vi "Periodic Message Filter.vi"(5 "Remove Immediately?(F)":bool, 7 "reset?":bool, 8 "Settings":T1={"threashold(#/s)"=1.0, "Check Peroid(s)"=1.0}, 11 "Cross CSM Data":T2={"Name(\"\" to use uuid)"="CSM Tiny", "Current State"="UI: Refresh Buttons", "Arguments"="", "Source Message"={"‘State"="", "’Arguments"="", "’Error"={"status"=FALSE, "code"=0, "source"=""}}, "Source Module"="<end>", "Complete(T)/Start(F)"=TRUE, "LogType"=enum."State Change"}) -> (0 "Boolean":bool, 1 "filter Strings Count":string[](array[string]), 3 "Log String":string)   [LabVIEW 2017, in "csm-tool-support.lvlib"]
uses:
  csm-tool-support.lvlib
  _Support/Typedef/_CSM_GlobalLog_MSG.ctl
  _Support/Typedef/_CSM_Response Source Message.ctl
  _Support/Typedef/_CSM_GlobalLog_MSG_TYPE.ctl
  Communicable State Machine.lvlib
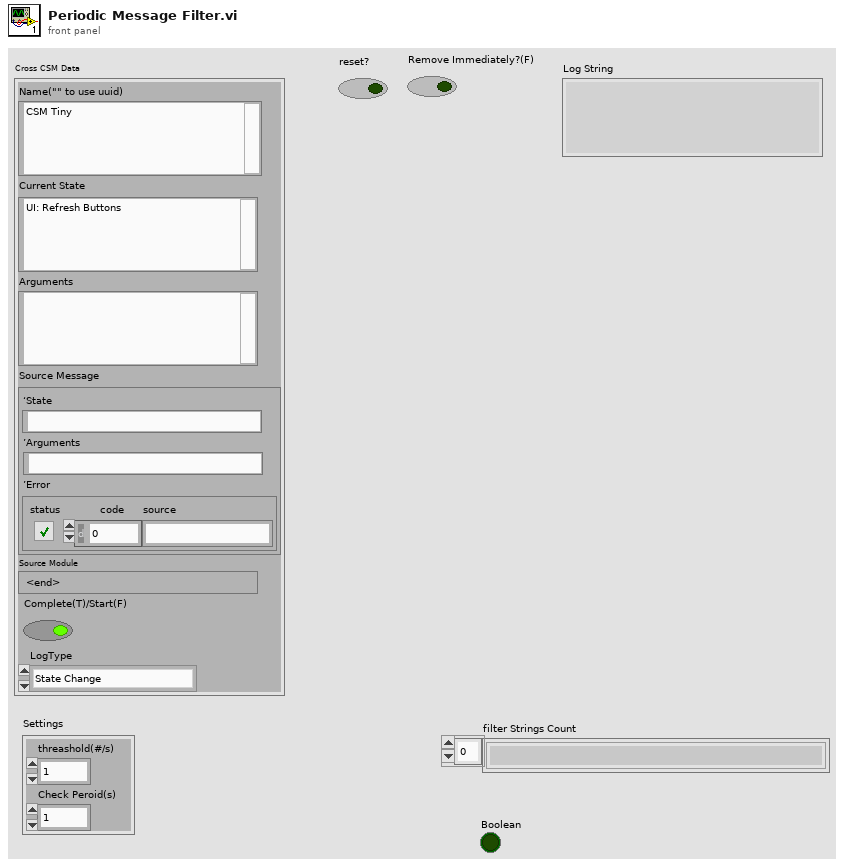
[diagram p1: front panel]
types:
  T1 = cluster{"threashold(#/s)":dbl, "Check Peroid(s)":dbl}
  T2 = typedef "Communicable State Machine.lvlib/_CSM_GlobalLog_MSG.ctl" = cluster{"Name(\"\" to use uuid)":string, "Current State":string, "Arguments":string, "Source Message":T3, "Source Module":string, "Complete(T)/Start(F)":bool, "LogType":T4}
  T3 = typedef "Communicable State Machine.lvlib/_CSM_Response Source Message.ctl" = cluster{"‘State":string, "’Arguments":string, "’Error":errorcluster}
  T4 = typedef "Communicable State Machine.lvlib/_CSM_GlobalLog_MSG_TYPE.ctl" = enum16{"User Log", "State Change", "Status", "Interrupt", "Register", "Unregister", "Error Log", "Module Created", "Module Destroyed"}
  T5 = cluster{"String":string, "Count":i64, "since":timestamp}[]
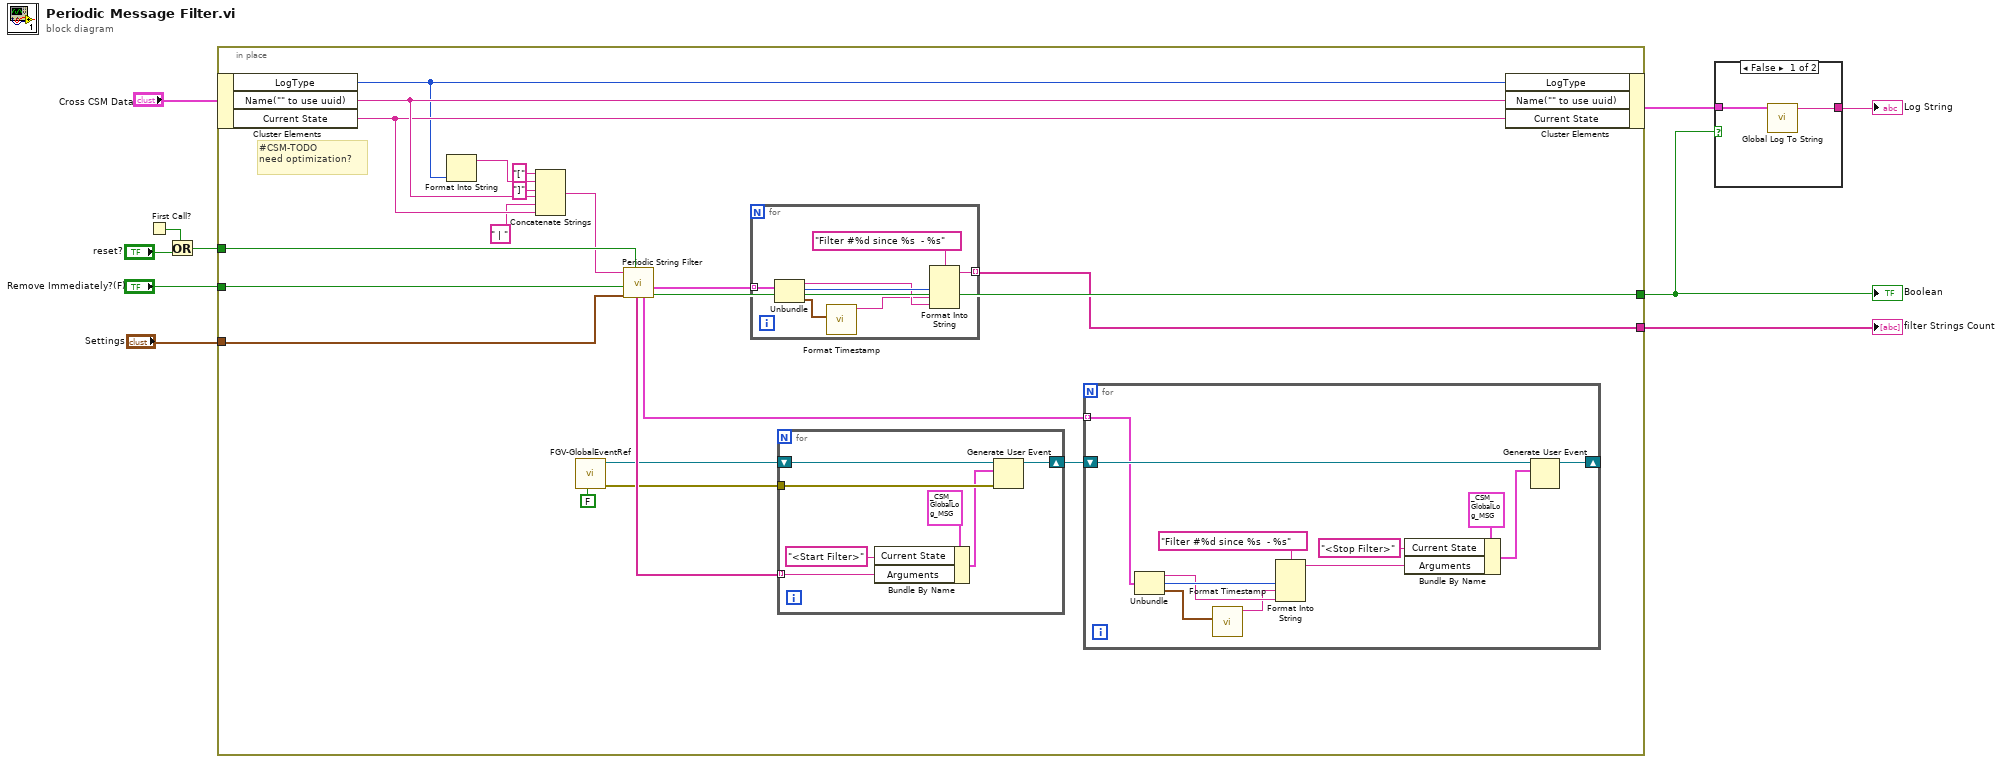
[diagram p0: block diagram]
diagram:
  n1 = First Call?() -> (First Call?: T/F=w7:bool)
  n2 = Or(x=w7, y="reset?") -> (x .or. y?=w5:bool)
  n3 = in-place {
    in-place-border: w5 -> [w25]
    in-place-border: [w23] -> w4
    in-place-border: [w19] -> w3
    in-place-border: "Remove Immediately?(F)" -> [w12]
    in-place-border: "Settings" -> [w11]
    # "#CSM-TODO\nneed optimization?"
    n4 = in-place-cluster #1("Cross CSM Data") -> ("LogType"=w28:T4, "Name(\"\" to use uuid)"=w30:string, "Current State"=w29:string)
    n5 = Format Into String(w28) -> (resulting string=w27:string)  [unwired: 3 in, 1 out]
    n6 = Concatenate Strings("[" ("string"), w27, "]" ("string"), w30, " | " ("string"), w29) -> (w24:string)
    n7 = call "FGV-GlobalEventRef.vi"("Create(F)"=FALSE) -> ("error out"=w15:errorcluster, "CSM Global Log Event"=w16:refnum<user-event>)  [unwired: 9 in]
    n8 = call "Periodic String Filter.vi"("reset?"=w25, "Settings"=w11, "Remove Immediately?(F)"=w12, "Input String"=w24) -> ("filtered?"=w23:bool, "Filtered Status"=w20:T5, "removed info"=w13:T5, "added Info"=w18:string[])  [unwired: 3 in, 1 out]
    n9 = for {
      tunnel: w20 -> [w55] mode=indexing
      tunnel: [w56] -> w19 mode=indexing
      n10 = Unbundle(w55) -> ("String"=w53:string, "Count"=w54:i64, "since"=w51:timestamp)
      n11 = call "Format Timestamp.vi"("timestamp"=w51) -> ("String"=w50:string)  [unwired: 10 in]
      n12 = Format Into String(format string="Filter #%d since %s  - %s", w54, w50, w53) -> (resulting string=w56:string)  [unwired: 2 in, 1 out]
    }
    n13 = for {
      tunnel: w18 -> [w44] mode=indexing
      tunnel: w15 -> [w48]
      shift-right: [w47] -> w14
      shift-left: w16 -> [w49]
      n14 = Bundle By Name(cluster=T2 {"Name(\"\" to use uuid)"="", "Current State"="", "Arguments"="", "Source Message"={"‘State"="", "’Arguments"="", "’Error"={"status"=FALSE, "code"=0, "source"=""}}, "Source Module"="", "Complete(T)/Start(F)"=FALSE, "LogType"=enum."User Log"} ("event data"), "Current State"="<Start Filter>", "Arguments"=w44) -> (w45:T2)
      n15 = Generate User Event(user event=w49, event data cluster=w45, error in=w48) -> (user event out=w47:refnum<user-event>)  [unwired: 1 in, 1 out]
    }
    n16 = for {
      shift-right: [w41] -> _
      shift-left: w14 -> [w42]
      tunnel: w13 -> [w37] mode=indexing
      n17 = Unbundle(w37) -> ("String"=w33:string, "Count"=w34:i64, "since"=w32:timestamp)
      n18 = call "Format Timestamp.vi"("timestamp"=w32) -> ("String"=w31:string)  [unwired: 10 in]
      n19 = Format Into String(format string="Filter #%d since %s  - %s", w34, w31, w33) -> (resulting string=w35:string)  [unwired: 2 in, 1 out]
      n20 = Bundle By Name(cluster=T2 {"Name(\"\" to use uuid)"="", "Current State"="", "Arguments"="", "Source Message"={"‘State"="", "’Arguments"="", "’Error"={"status"=FALSE, "code"=0, "source"=""}}, "Source Module"="", "Complete(T)/Start(F)"=FALSE, "LogType"=enum."User Log"} ("event data"), "Current State"="<Stop Filter>", "Arguments"=w35) -> (w38:T2)
      n21 = Generate User Event(user event=w42, event data cluster=w38) -> (user event out=w41:refnum<user-event>)  [unwired: 2 in, 1 out]
    }
    n22 = in-place-cluster #1("LogType"=w28, "Name(\"\" to use uuid)"=w30, "Current State"=w29) -> (w9:T2)
  }
  "Boolean" <- w4
  "filter Strings Count" <- w3
  n23 = case shown="False" w4 {
    tunnel: [w58 _] -> w8
    tunnel: w9 -> [w57 _]
    frame False {
      n24 = call "Global Log To String.vi"("Log"=w57) -> ("Log String"=w58:string)  [unwired: 9 in]
    }
    frame True {
    }
  }
  "Log String" <- w8
